vi "limelight-turret_converter.vi"(2 "VisionTarget":T1, 3 "Limelight Radius (in)":dbl) -> (0 "Turret Yaw Angle (deg)":dbl, 1 "Turret Distance (in)":dbl)   [LabVIEW 2019]
uses:
  TypeDefs/VisionTarget.ctl
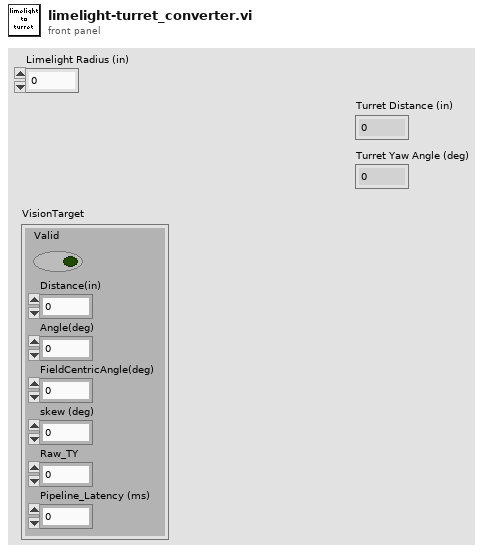
[diagram p1: front panel]
types:
  T1 = typedef "VisionTarget.ctl" = cluster{"Valid":bool, "Distance(in)":dbl, "Angle(deg)":dbl, "FieldCentricAngle(deg)":dbl, "skew (deg)":dbl, "Raw_TY":dbl, "Pipeline_Latency (ms)":dbl}
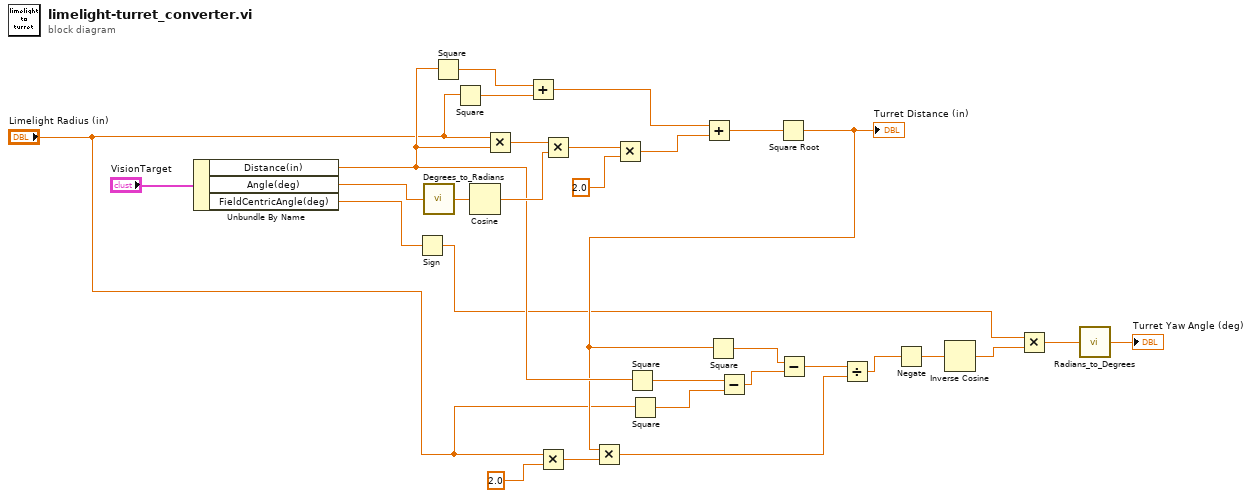
[diagram p0: block diagram]
diagram:
  n1 = Unbundle By Name("VisionTarget") -> ("Distance(in)"=w14:dbl, "Angle(deg)"=w29:dbl, "FieldCentricAngle(deg)"=w18:dbl)
  n2 = Sign(1:w18) -> (0:w3:dbl)
  n3 = call "Degrees_to_Radians.vi"("Degrees"=w29) -> ("Radians"=w28:dbl)
  n4 = Square(x=w14) -> (x^2=w22:dbl)
  n5 = Square(x="Limelight Radius (in)") -> (x^2=w23:dbl)
  n6 = Cosine(x=w28) -> (cos(x)=w27:dbl)
  n7 = Multiply(x="Limelight Radius (in)", y=w14) -> (x*y=w26:dbl)
  n8 = Add(x=w22, y=w23) -> (x+y=w21:dbl)
  n9 = Multiply(x="Limelight Radius (in)", y=2.0) -> (x*y=w16:dbl)
  n10 = Multiply(x=w26, y=w27) -> (x*y=w24:dbl)
  n11 = Multiply(x=w24, y=2.0) -> (x*y=w20:dbl)
  n12 = Square(x=w14) -> (x^2=w13:dbl)
  n13 = Square(x="Limelight Radius (in)") -> (x^2=w12:dbl)
  n14 = Add(x=w21, y=w20) -> (x+y=w19:dbl)
  n15 = Subtract(x=w13, y=w12) -> (x-y=w7:dbl)
  n16 = Square Root(x=w19) -> (sqrt(x)=w10:dbl)
  "Turret Distance (in)" <- w10
  n17 = Multiply(x=w10, y=w16) -> (x*y=w15:dbl)
  n18 = Square(x=w10) -> (x^2=w8:dbl)
  n19 = Subtract(x=w8, y=w7) -> (x-y=w9:dbl)
  n20 = Divide(x=w9, y=w15) -> (x/y=w6:dbl)
  n21 = Negate(x=w6) -> (-x=w5:dbl)
  n22 = Inverse Cosine(1:w5) -> (0:w4:dbl)
  n23 = Multiply(x=w3, y=w4) -> (x*y=w2:dbl)
  n24 = call "Radians_to_Degrees.vi"("Radians"=w2) -> ("Degrees"=→"Turret Yaw Angle (deg)":dbl)
